vi "Refresh Indicators.vi"(8 "error in (no error)":errorcluster, 11 "PluginGUI in":refnum<class "PluginGUI.lvclass">) -> (0 "error out":errorcluster, 3 "PluginGUI out":refnum<class "PluginGUI.lvclass">)   [LabVIEW 2020, in "VolatusGUI.lvlib" / "PluginGUI.lvclass"]
uses:
  PluginGUI.lvclass
  PluginGUI.lvclass/PluginGUI.ctl
  GUI Element/GUI Element.lvclass
  Indicator/Indicator.lvclass
  C:/dev/lv20CE/relink/lv-volatus/VolatusGUI/GUI Element/GUI Element.lvclass
  C:/dev/lv20CE/relink/lv-volatus/VolatusGUI/Indicator/Indicator.lvclass
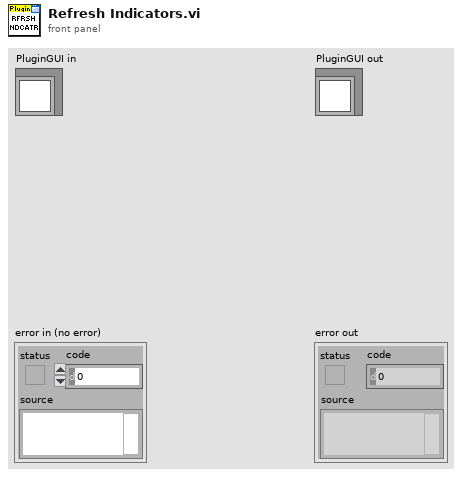
[diagram p1: front panel]
types:
  T1 = map{refnum<vi>, refnum<class "Indicator.lvclass">}
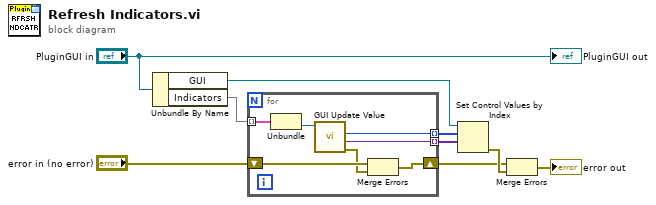
[diagram p0: block diagram]
diagram:
  n1 = Unbundle By Name("PluginGUI in") -> ("GUI"=w5:refnum<vi>, "Indicators"=w8:T1)
  n2 = for {
    tunnel: w8 -> [w16] mode=indexing
    tunnel: [w14] -> w7 mode=indexing
    tunnel: [w13] -> w6 mode=indexing
    shift-right: [w10] -> w2
    shift-left: "error in (no error)" -> [w12]
    n3 = Unbundle(w16) -> ("Indicator"=w15:refnum<class "Indicator.lvclass">)  [unwired: 1 out]
    n4 = call "GUI Update Value.vi"("GUI Element in"=w15) -> ("error out"=w11:errorcluster, "Value"=w13:variant, "Control Index"=w14:i32)  [unwired: 7 in, 1 out]
    n5 = Merge Errors(w12, w11) -> (w10:errorcluster)
  }
  n6 = Set Control Values by Index(0:w5, 1:w7, 2:w6) -> (11:w3:errorcluster)  [unwired: 1 in]
  n7 = Merge Errors(w2, w3) -> (→"error out":errorcluster)
  "PluginGUI out" <- "PluginGUI in"
